vi "_35_Sample_qsns_9[11].vi"() -> ()   [LabVIEW 2020]
panel:
  out "x .xor. y?":i32
  out "x+1":dbl
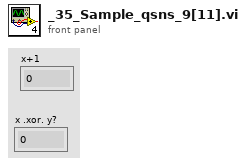
[diagram p1: front panel]
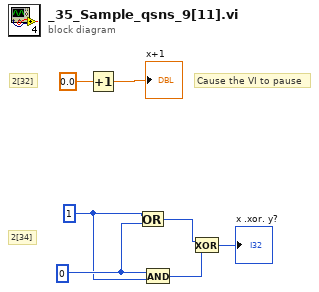
[diagram p0: block diagram]
diagram:
  w3 = 0
  w2 = 1
  # "2[34]"
  # "Cause the VI to pause"
  # "2[32]"
  n1 = Increment(x=0.0) -> (x+1=→"x+1":dbl)
  n2 = Or(x=w2, y=w3) -> (x .or. y?=w5:i32)
  n3 = And(x=w3, y=w2) -> (x .and. y?=w4:i32)
  n4 = Exclusive Or(1:w4, 2:w5) -> (0:→"x .xor. y?":i32)
